vi "F2V Basic.vi"(11 "ForceArray In":fxp<+/-,25,5>[](array[numeric])=[0.0, 0.0, 0.0, 0.0, 0.0]) -> (3 "ElectrodeVoltageArray Out":fxp<+/-,20,5>[](array[numeric]))   [LabVIEW 2020, in "CtrlEff.lvlib" / "Force2Volt.lvlib"]
doc: "Convert actuation forces into electrode voltages with the appropriate sign.\nBasic version: just pass the force values with appropriate signs."
uses:
  Force2Volt.lvlib
  <vilib>/Platform/TimedLoop/XDataNode/timing_clust.ctl
  <vilib>/Platform/TimedLoop/XDataNode/nitl_modes.ctl
  <vilib>/Platform/TimedLoop/XDataNode/wakeup.ctl
  <vilib>/rvi/Emulation/niFpgaSctlEmulationGetInTimedLoop.vi
  <vilib>/rvi/Emulation/niFpgaEmulationReportErrorSimple.vi
  <vilib>/rvi/Emulation/niFpgaGetClockAttributes.vi
  <vilib>/rvi/Emulation/niFpgaCriticalErrorInLSC.vi
  <vilib>/Platform/TimedLoop/XDataNode/XDataNode.xnode
  <vilib>/Platform/TimedLoop/XDataNode/XDNodeRunTimeDep.lvlib
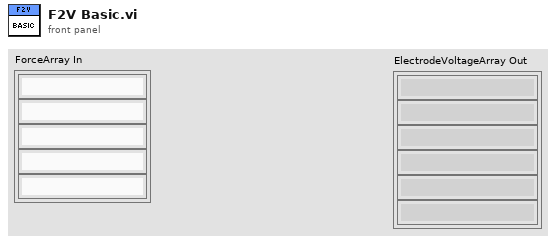
[diagram p1: front panel]
types:
  T1 = typedef "XDNodeRunTimeDep.lvlib/timing_clust.ctl" = cluster{"Expected End [f-1]":u64, "Actual End [f-1]":u64, "Finished Late? [f-1]":bool, "Expected End [i-1]":u64, "Actual End [i-1]":u64, "Finished Late? [i-1]":bool, "Expected Start [i]":u64, "Actual Start [i]":u64, "Expected Start [f]":u64, "Actual Start [f]":u64, "Source Name":string, "Structure Name":string, "Period":i64, "Deadline":i64, "Offset":i64, "Start":i64, "Priority":i32, "Timeout":i32, "Mode":T2, "Wakeup Reason":T3, "Error":errorcluster, "Source Type":string, "Secondary Source Type":string, "Global End Time":u64, "Global Start Time":u64, "Frame Duration":u64, "Iteration Duration":u64, "Assigned CPU":i32, "I/O Scan Engine Mode":u32}
  T2 = typedef "XDNodeRunTimeDep.lvlib/nitl_modes.ctl" = enum32{"No Change", "Process missed periods, maintain original phase", "Discard missed periods, maintain original phase", "Process missed periods, ignore original phase", "Discard missed periods, ignore original phase"}
  T3 = typedef "XDNodeRunTimeDep.lvlib/wakeup.ctl" = enum32{"Normal", "Aborted", "Asynchronous wakeup", "Timing source error", "Timed loop error", "Timeout"}
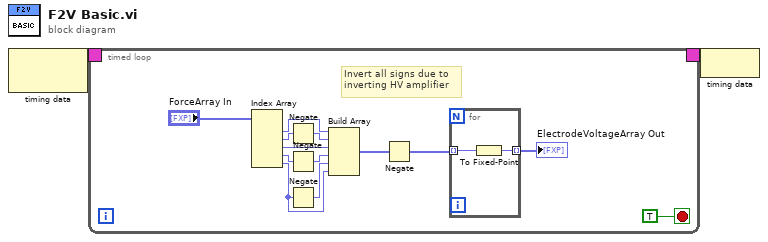
[diagram p0: block diagram]
diagram:
  n1 = node-c288() -> (w2:T1)  [unwired: 1 in]
  n2 = timed-loop {
    timing: w2 -> [_]
    timing-out: [_] -> w1
    stop <- TRUE stop-if-true
    # "Invert all signs due to \ninverting HV amplifier"
    n3 = Index Array(array="ForceArray In") -> (element #1=w14:fxp<+/-,25,5>, element #2=w13:fxp<+/-,25,5>, element #3=w11:fxp<+/-,25,5>, element #4=w10:fxp<+/-,25,5>, element #5=w7:fxp<+/-,25,5>)  [unwired: 5 in]
    n4 = Negate(x=w13) -> (-x=w12:fxp<+/-,26,6>)
    n5 = Negate(x=w10) -> (-x=w9:fxp<+/-,26,6>)
    n6 = Negate(x=w7) -> (-x=w8:fxp<+/-,26,6>)
    n7 = Build Array(w14, w12, w11, w9, w8, w7) -> (w4:fxp<+/-,26,6>[])
    n8 = Negate(x=w4) -> (-x=w3:fxp<+/-,26,6>[])
    n9 = for {
      tunnel: w3 -> [w17] mode=indexing
      tunnel: [w16] -> w6 mode=indexing
      n10 = To Fixed-Point(number=w17) -> (fixed-point=w16:fxp<+/-,20,5>)  [unwired: 1 in]
    }
    "ElectrodeVoltageArray Out" <- w6
  }
  n11 = node-c288(w1) -> ()
